vi "Run Tx - Timed RT.vi"(7 "Process in":refnum<class "Process.lvclass">, 8 "error in (no error)":errorcluster, 11 "Tx Loop Data in":T1) -> (3 "Tx Loop Data out":T1)   [LabVIEW 2021, in "UDP-Custom-Device Engine.lvlib"]
uses:
  UDP-Custom-Device Engine.lvlib
  <vilib>/NI/NIVS Inline Async API/_VS Inline Async API/Process/Process.lvclass
  Types/Engine - Tx Loop Data.ctl
  <vilib>/NI VeriStand/VeriStand Data/Byte Buffer/Byte Buffer.lvclass
  Types/Engine - General Resources.ctl
  <vilib>/NI VeriStand/VeriStand Data/Typedefs/Typedefs.Data Types.ctl
  Shared/Types/Shared - Duplex Settings.ctl
  Shared/Types/Shared - Header Details.ctl
  Types/Engine - Data Conversion Config.ctl
  <vilib>/NI VeriStand/VeriStand Data/Byte Buffer/Byte Buffer.Mapping.ctl
  Types/Engine - Tx Runtime Resources.ctl
  Shared/Types/Shared - Transmit Flag Options.ctl
  Types/Engine - Execution Config.ctl
  Shared/Types/Shared - Thread Management.ctl
  Types/Engine - Tx Echo Resources.ctl
  Shared/Types/Shared - Transmit Echo Options.ctl
  Types/Engine - Tx Channel Refs.ctl
  <vilib>/NI/NIVS Inline Async API/_Data Access Engine/Data Access Engine/Types/Read.DVR.ctl
  <vilib>/NI/NIVS Inline Async API/_Data Access Engine/Access Type Classes/Read/Read.lvclass
  <vilib>/NI/NIVS Inline Async API/_Data Access Engine/Data Access Engine/Types/Write.DVR.ctl
  <vilib>/NI/NIVS Inline Async API/_Data Access Engine/Access Type Classes/Write/Write.lvclass
  Types/Engine - Debug Resources.ctl
  <vilib>/Platform/TimedLoop/XDataNode/timing_clust.ctl
  <vilib>/Platform/TimedLoop/XDataNode/nitl_modes.ctl
  <vilib>/Platform/TimedLoop/XDataNode/wakeup.ctl
  <vilib>/NI/NIVS Inline Async API/_Data Access Engine/Access Type Classes/Read/Read.lvclass/Read.ctl
  <vilib>/NI VeriStand/VeriStand Data/Byte Buffer/Byte Buffer.lvclass/Byte Buffer.ctl
  <vilib>/NI/NIVS Inline Async API/_Data Access Engine/Access Type Classes/Write/Write.lvclass/Write.ctl
  <vilib>/NI/NIVS Inline Async API/_VS Inline Async API/Process/Process.lvclass/Process.ctl
  <vilib>/NI/NIVS Inline Async API/_VS Inline Async API/Error Handling Process/SubVIs/Error.ConvertArray.vi
  Run Tx - Handle Transmit Option.vi
  Run Tx - Handle Port Tx Check.vi
  <vilib>/NI/NIVS Inline Async API/_Data Access Engine/Data Access Engine/Methods/Data.Processes.Execute.vi
  <vilib>/NI/NIVS Inline Async API/_Data Access Engine/Data Access Engine/Methods/Write.Data.vi
  <vilib>/NI/NIVS Inline Async API/_Data Access Engine/Data Access Engine/Methods/Read.Data.vi
  Tx to UDP.vi
  <vilib>/NI/NIVS Inline Async API/_Data Access Engine/Access Type Classes/Write/Write.ProcessData.vi
  <vilib>/NI/NIVS Inline Async API/_Data Access Engine/Access Type Classes/Read/Read.ProcessData.vi
  <vilib>/NI VeriStand/VeriStand Data/Byte Buffer/Byte Buffer.Mapping.Write.vi
  <vilib>/NI VeriStand/VeriStand Data/Pointer Operations/Pointer.Write.vi
  <vilib>/NI VeriStand/VeriStand Data/Pointer Operations/Pointer.Write (DBL).vi
  <vilib>/NI VeriStand/VeriStand Data/Byte Buffer/Byte Buffer.Read.vi
  <vilib>/NI VeriStand/VeriStand Data/Byte Buffer/Byte Buffer.Read (String).vi
  <vilib>/NI VeriStand/VeriStand Data/Byte Buffer/Byte Buffer.Get Buffer Size.vi
  <vilib>/NI/NIVS Inline Async API/_Data Access Engine/Access Type Classes/Write/Write.Buffer.vi
  <vilib>/NI/NIVS Inline Async API/_Data Access Engine/Access Type Classes/Write/Write.Commit.vi
  <vilib>/NI VeriStand/VeriStand Data/Memory Management/Memory Management.MoveDblBlock.Write (Double).vi
  <vilib>/NI VeriStand/VeriStand Data/Byte Buffer/Byte Buffer.Write.Typed Double Array.vi
  <vilib>/NI VeriStand/VeriStand Data/Utilities/Utilities.Buffer.Double.vi
  <vilib>/NI VeriStand/VeriStand Data/Byte Buffer/Byte Buffer.Subset.Get.vi
  <vilib>/NI VeriStand/VeriStand Data/Byte Buffer/Byte Buffer.Write.vi
  <vilib>/NI VeriStand/VeriStand Data/Byte Buffer/Byte Buffer.Write (1D Boolean).vi
  <vilib>/NI VeriStand/VeriStand Data/Type Conversion/Type Conversion.From Double.Subset.vi
  <vilib>/NI VeriStand/VeriStand Data/Type Conversion/Type Conversion.From Double.Subset (1D Boolean).vi
  <vilib>/NI VeriStand/VeriStand Data/Byte Buffer/Byte Buffer.Write (1D SGL).vi
  <vilib>/NI VeriStand/VeriStand Data/Type Conversion/Type Conversion.From Double.Subset (1D SGL).vi
  <vilib>/NI VeriStand/VeriStand Data/Byte Buffer/Byte Buffer.Write (1D DBL).vi
  <vilib>/NI VeriStand/VeriStand Data/Byte Buffer/Byte Buffer.Write (1D I8).vi
  <vilib>/NI VeriStand/VeriStand Data/Type Conversion/Type Conversion.From Double.Subset (1D I8).vi
  <vilib>/NI VeriStand/VeriStand Data/Byte Buffer/Byte Buffer.Write (1D I16).vi
  <vilib>/NI VeriStand/VeriStand Data/Type Conversion/Type Conversion.From Double.Subset (1D I16).vi
  <vilib>/NI VeriStand/VeriStand Data/Byte Buffer/Byte Buffer.Write (1D I32).vi
  <vilib>/NI VeriStand/VeriStand Data/Type Conversion/Type Conversion.From Double.Subset (1D I32).vi
  <vilib>/NI VeriStand/VeriStand Data/Byte Buffer/Byte Buffer.Write (1D I64).vi
  <vilib>/NI VeriStand/VeriStand Data/Type Conversion/Type Conversion.From Double.Subset (1D I64).vi
  <vilib>/NI VeriStand/VeriStand Data/Byte Buffer/Byte Buffer.Write (1D U8).vi
  <vilib>/NI VeriStand/VeriStand Data/Type Conversion/Type Conversion.From Double.Subset (1D U8).vi
  <vilib>/NI VeriStand/VeriStand Data/Byte Buffer/Byte Buffer.Write (1D U16).vi
  <vilib>/NI VeriStand/VeriStand Data/Type Conversion/Type Conversion.From Double.Subset (1D U16).vi
  <vilib>/NI VeriStand/VeriStand Data/Byte Buffer/Byte Buffer.Write (1D U32).vi
  <vilib>/NI VeriStand/VeriStand Data/Type Conversion/Type Conversion.From Double.Subset (1D U32).vi
  <vilib>/NI VeriStand/VeriStand Data/Byte Buffer/Byte Buffer.Write (1D U64).vi
  <vilib>/NI VeriStand/VeriStand Data/Type Conversion/Type Conversion.From Double.Subset (1D U64).vi
  <vilib>/NI VeriStand/VeriStand Data/Memory Management/Memory Management.MoveByteBlock.Write (String).vi
  <vilib>/NI VeriStand/VeriStand Data/Byte Buffer/Byte Buffer.Get Buffer Pointer.vi
  <vilib>/NI VeriStand/VeriStand Data/Byte Buffer/Byte Buffer.Write (String).vi
  <vilib>/NI VeriStand/VeriStand Data/Type Conversion/Type Conversion.From Double.vi
  <vilib>/NI VeriStand/VeriStand Data/Type Conversion/Type Conversion.From Double (1D Boolean).vi
  <vilib>/NI VeriStand/VeriStand Data/Type Conversion/Type Conversion.From Double (1D SGL).vi
  <vilib>/NI VeriStand/VeriStand Data/Type Conversion/Type Conversion.From Double (1D I8).vi
  <vilib>/NI VeriStand/VeriStand Data/Type Conversion/Type Conversion.From Double (1D I16).vi
  <vilib>/NI VeriStand/VeriStand Data/Type Conversion/Type Conversion.From Double (1D I32).vi
  <vilib>/NI VeriStand/VeriStand Data/Type Conversion/Type Conversion.From Double (1D I64).vi
  <vilib>/NI VeriStand/VeriStand Data/Type Conversion/Type Conversion.From Double (1D U8).vi
  <vilib>/NI VeriStand/VeriStand Data/Type Conversion/Type Conversion.From Double (1D U16).vi
  <vilib>/NI VeriStand/VeriStand Data/Type Conversion/Type Conversion.From Double (1D U32).vi
  <vilib>/NI VeriStand/VeriStand Data/Type Conversion/Type Conversion.From Double (1D U64).vi
  <vilib>/NI VeriStand/VeriStand Data/Byte Buffer/Byte Buffer.Subset.Set.vi
  <vilib>/NI VeriStand/VeriStand Data/Memory Management/Memory Management.MoveByteBlock.Read (String).vi
  <vilib>/NI VeriStand/VeriStand Data/Memory Management/Memory Management.Handle Return.vi
  <vilib>/NI VeriStand/VeriStand Data/Byte Buffer/Byte Buffer.Get Byte Order.vi
  <vilib>/platform/TimedLoop/XDataNode/XDataNode.xnode
  <vilib>/Platform/TimedLoop/XDataNode/XDNodeRunTimeDep.lvlib
  <vilib>/NI VeriStand/VeriStand Data/VeriStand Data.lvlib
  Shared/UDP-Custom-Device Shared.lvlib
  <vilib>/NI/NIVS Inline Async API/_Data Access Engine/Data Access Engine/Data Access Engine.lvclass
panel:
  out "length":i32
  out "Tx Packet":string
  # "CHANNEL TRANSMIT\n- TIMED\n- REALTIME ONLY"
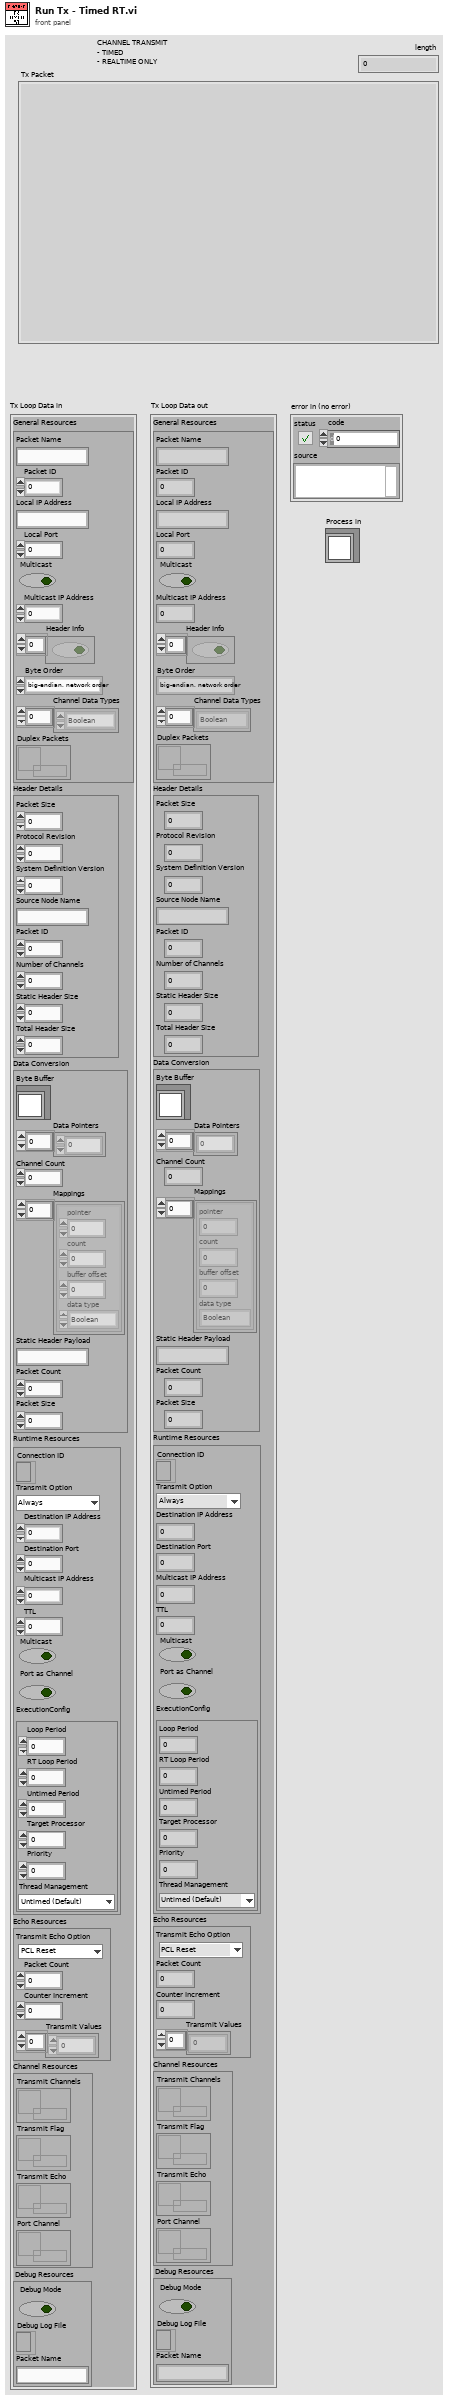
[diagram p1: front panel]
types:
  T1 = typedef "UDP-Custom-Device Engine.lvlib/Engine - Tx Loop Data.ctl" = cluster{"General Resources":T2, "Header Details":T4, "Data Conversion":T5, "Runtime Resources":T7, "Echo Resources":T11, "Channel Resources":T13, "Debug Resources":T16}
  T2 = typedef "UDP-Custom-Device Engine.lvlib/Engine - General Resources.ctl" = cluster{"Packet Name":string, "Packet ID":i32, "Local IP Address":string, "Local Port":i32, "Multicast":bool, "Multicast IP Address":u32, "Header Info":bool[], "Byte Order":enum16{"big-endian, network order", "native, host order", "little-endian"}, "Channel Data Types":T3[], "Duplex Packets":refnum<data-value>}
  T3 = typedef "VeriStand Data.lvlib/Typedefs.Data Types.ctl" = enum16{"Boolean", "Single", "Double", "I8", "I16", "I32", "I64", "U8", "U16", "U32", "U64"}
  T4 = typedef "UDP-Custom-Device Shared.lvlib/Shared - Header Details.ctl" = cluster{"Packet Size":u16, "Protocol Revision":u8, "System Definition Version":u64, "Source Node Name":string, "Packet ID":u32, "Number of Channels":u32, "Static Header Size":u16, "Total Header Size":u16}
  T5 = typedef "UDP-Custom-Device Engine.lvlib/Engine - Data Conversion Config.ctl" = cluster{"Byte Buffer":refnum<class "Byte Buffer.lvclass">, "Data Pointers":u64[], "Channel Count":i32, "Mappings":T6[], "Static Header Payload":string, "Packet Count":dbl, "Packet Size":i32}
  T6 = typedef "VeriStand Data.lvlib/Byte Buffer.lvclass/Byte Buffer.Mapping.ctl" = cluster{"pointer":u64, "count":i64, "buffer offset":u64, "data type":T3}
  T7 = typedef "UDP-Custom-Device Engine.lvlib/Engine - Tx Runtime Resources.ctl" = cluster{"Connection ID":refnum<k16>, "Transmit Option":T8, "Destination IP Address":u32, "Destination Port":u16, "Multicast IP Address":u32, "TTL":u16, "Multicast":bool, "Port as Channel":bool, "ExecutionConfig":T9}
  T8 = typedef "UDP-Custom-Device Shared.lvlib/Shared - Transmit Flag Options.ctl" = enum16{"Always", "One-Shot", "Toggle"}
  T9 = typedef "UDP-Custom-Device Engine.lvlib/Engine - Execution Config.ctl" = cluster{"Loop Period":i64, "RT Loop Period":i64, "Untimed Period":u32, "Target Processor":i32, "Priority":i32, "Thread Management":T10}
  T10 = typedef "UDP-Custom-Device Shared.lvlib/Shared - Thread Management.ctl" = enum16{"Untimed (Default)", "Timed (High Priority)"}
  T11 = typedef "UDP-Custom-Device Engine.lvlib/Engine - Tx Echo Resources.ctl" = cluster{"Transmit Echo Option":T12, "Packet Count":dbl, "Counter Increment":dbl, "Transmit Values":dbl[]}
  T12 = typedef "UDP-Custom-Device Shared.lvlib/Shared - Transmit Echo Options.ctl" = enum16{"PCL Reset", "Counter", "Mirror"}
  T13 = typedef "UDP-Custom-Device Engine.lvlib/Engine - Tx Channel Refs.ctl" = cluster{"Transmit Channels":T14, "Transmit Flag":T14, "Transmit Echo":T15, "Port Channel":T14}
  T14 = typedef "Data Access Engine.lvlib/Data Access Engine.lvclass/Read.DVR.ctl" = refnum<data-value>
  T15 = typedef "Data Access Engine.lvlib/Data Access Engine.lvclass/Write.DVR.ctl" = refnum<data-value>
  T16 = typedef "UDP-Custom-Device Engine.lvlib/Engine - Debug Resources.ctl" = cluster{"Debug Mode":bool, "Debug Log File":refnum<file>, "Packet Name":string}
  T17 = typedef "XDNodeRunTimeDep.lvlib/timing_clust.ctl" = cluster{"Expected End [f-1]":u64, "Actual End [f-1]":u64, "Finished Late? [f-1]":bool, "Expected End [i-1]":u64, "Actual End [i-1]":u64, "Finished Late? [i-1]":bool, "Expected Start [i]":u64, "Actual Start [i]":u64, "Expected Start [f]":u64, "Actual Start [f]":u64, "Source Name":string, "Structure Name":string, "Period":i64, "Deadline":i64, "Offset":i64, "Start":i64, "Priority":i32, "Timeout":i32, "Mode":T18, "Wakeup Reason":T19, "Error":errorcluster, "Source Type":string, "Secondary Source Type":string, "Global End Time":u64, "Global Start Time":u64, "Frame Duration":u64, "Iteration Duration":u64, "Assigned CPU":i32, "I/O Scan Engine Mode":u32}
  T18 = typedef "XDNodeRunTimeDep.lvlib/nitl_modes.ctl" = enum32{"No Change", "Process missed periods, maintain original phase", "Discard missed periods, maintain original phase", "Process missed periods, ignore original phase", "Discard missed periods, ignore original phase"}
  T19 = typedef "XDNodeRunTimeDep.lvlib/wakeup.ctl" = enum32{"Normal", "Aborted", "Asynchronous wakeup", "Timing source error", "Timed loop error", "Timeout"}
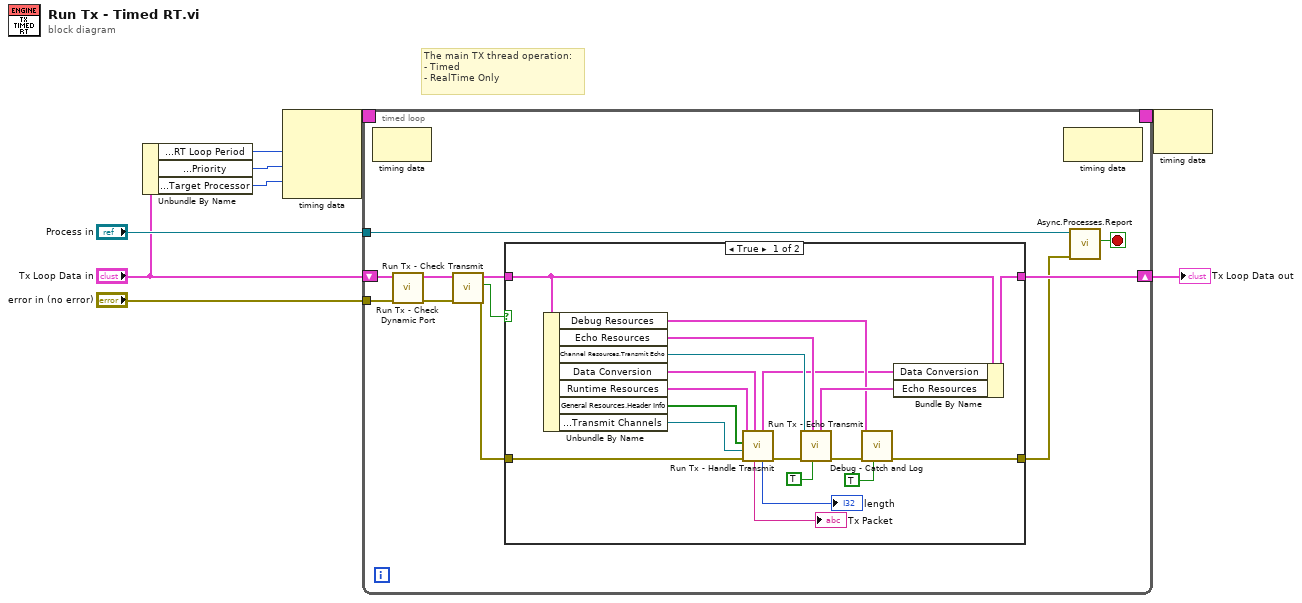
[diagram p0: block diagram]
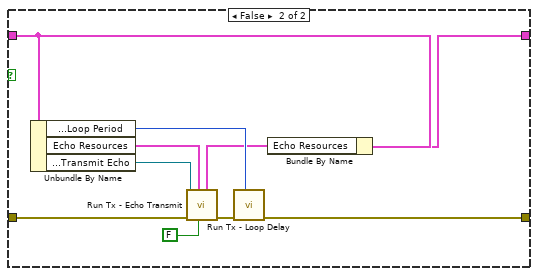
[diagram p2: hidden frame]
diagram:
  # "The main TX thread operation:\n- Timed\n- RealTime Only"
  n1 = Unbundle By Name("Tx Loop Data in") -> ("Runtime Resources.ExecutionConfig.RT Loop Period"=w7:i64, "Runtime Resources.ExecutionConfig.Priority"=w6:i32, "Runtime Resources.ExecutionConfig.Target Processor"=w5:i32)
  n2 = node-c288(w7, w6, w5) -> (w9:T17)  [unwired: 1 in]
  n3 = timed-loop {
    tunnel: "error in (no error)" -> [w10]
    tunnel: "Process in" -> [w20]
    shift-right: [w18] -> w2
    shift-left: "Tx Loop Data in" -> [w13]
    timing: w9 -> [_]
    timing-out: [_] -> w8
    stop <- w19 stop-if-true
    n4 = node-c288() -> ()  [unwired: 1 in, 1 out]
    n5 = call "Run Tx - Check Dynamic Port.vi"("error in (no error)"=w10, "Tx Loop Data in"=w13) -> ("error out"=w11:errorcluster, "Tx Loop Data out"=w12:T1)  [unwired: 8 in]
    n6 = call "Run Tx - Check Transmit.vi"("error in (no error)"=w11, "Tx Loop Data in"=w12) -> ("error out"=w16:errorcluster, "Transmit?"=w15:bool, "Tx Loop Data out"=w17:T1)  [unwired: 7 in]
    n7 = case shown="True" w15 {
      tunnel: [w35 w47] -> w14
      tunnel: [w41 w43] -> w18
      tunnel: w17 -> [w40 w44]
      tunnel: w16 -> [w27 w50]
      frame True {
        n8 = Unbundle By Name(w40) -> ("Debug Resources"=w33:T16, "Echo Resources"=w38:T11, "Channel Resources.Transmit Echo"=w39:T15, "Data Conversion"=w32:T5, "Runtime Resources"=w30:T7, "General Resources.Header Info"=w29:bool[], "Channel Resources.Transmit Channels"=w28:T14)
        n9 = call "Run Tx - Handle Transmit.vi"("Data Conversion"=w32, "error in (no error)"=w27, "Transmit Chanels"=w28, "Header Info"=w29, "Runtime Resources"=w30) -> ("error out"=w26:errorcluster, "length"=→"length":i32, "Data Conversion out"=w31:T5, "Tx Packet"=→"Tx Packet":string)  [unwired: 3 in]
        n10 = call "Run Tx - Echo Transmit.vi"("Transmitted?"=TRUE, "Echo Resources in"=w38, "error in (no error)"=w26, "Ref"=w39) -> ("error out"=w25:errorcluster, "Echo Resources out"=w37:T11)  [unwired: 6 in]
        n11 = call "Debug - Catch and Log.vi"("Clear Error?"=TRUE, "error in (no error)"=w25, "Debug Resources"=w33) -> ("error out"=w35:errorcluster)  [unwired: 8 in]
        n12 = Bundle By Name(cluster=w40, "Data Conversion"=w31, "Echo Resources"=w37) -> (w41:T1)
      }
      frame False {
        n13 = Unbundle By Name(w44) -> ("Runtime Resources.ExecutionConfig.Loop Period"=w49:i64, "Echo Resources"=w45:T11, "Channel Resources.Transmit Echo"=w51:T15)
        n14 = call "Run Tx - Echo Transmit.vi"("Transmitted?"=FALSE, "Echo Resources in"=w45, "error in (no error)"=w50, "Ref"=w51) -> ("error out"=w48:errorcluster, "Echo Resources out"=w42:T11)  [unwired: 6 in]
        n15 = call "Run Tx - Loop Delay.vi"("Delay (ms)"=w49, "error in (no error)"=w48) -> ("error out"=w47:errorcluster)  [unwired: 9 in]
        n16 = Bundle By Name(cluster=w44, "Echo Resources"=w42) -> (w43:T1)
      }
    }
    n17 = node-c288() -> ()  [unwired: 1 in, 1 out]
    n18 = call <vilib>:"Async.Processes.Report.vi"("Error"=w14, "Process in"=w20) -> ("Stop"=w19:bool)  [unwired: 8 in, 1 out]
  }
  "Tx Loop Data out" <- w2
  n19 = node-c288(w8) -> ()  [unwired: 1 out]
